vi "Teleop.vi"(10 "Match Info":T1={"Autonomous Elapsed Seconds"=0.0, "TeleOp Elapsed Seconds"=0.0, "Disabled Elapsed Seconds"=0.0, "Visited Autonomous"=FALSE, "Visited TeleOp"=FALSE, "Visited Disabled"=FALSE, "Autonomous Settings"={"Autonomous Style"=enum."Independent", "VI Refnum"=refnum}}, 11 "Call Context":T2) -> ()   [LabVIEW 2019]
doc: "This VI is called for each TeleOp packet received from the DS where the robot is not disabled. It is often used to read from the joysticks and update I/O or to update setpoints for timed control loops. It should complete and return within 20 milliseconds or it may miss DS packets."
uses:
  <vilib>/Rock Robotics/WPI/DriverStation/WPI_DriverStationDerivedRobotMode.ctl
  <vilib>/Rock Robotics/WPI/DriverStation/WPI_DriverStationMatch Info.ctl
  <vilib>/Rock Robotics/WPI/Utilities/WPI_GetSetVariantRefNum.vi
  <vilib>/Rock Robotics/Network Tables/NT Write Boolean Array.vi
  <vilib>/Rock Robotics/Network Tables/NT Write Numeric Array.vi
  <vilib>/Rock Robotics/Network Tables/NT Write Number.vi
  <vilib>/Rock Robotics/WPI/RobotDrive/WPI_RobotDriveMecanumDrive_Cartesian.vi
  <vilib>/Rock Robotics/WPI/RobotDrive/WPI_RobotDriveMecanumDrive_Polar.vi
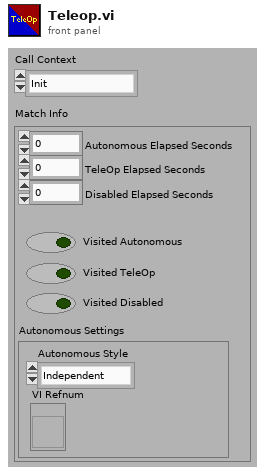
[diagram p1: front panel]
types:
  T1 = typedef "WPI_DriverStationMatch Info.ctl" = cluster{"Autonomous Elapsed Seconds":dbl, "TeleOp Elapsed Seconds":dbl, "Disabled Elapsed Seconds":dbl, "Visited Autonomous":bool, "Visited TeleOp":bool, "Visited Disabled":bool, "Autonomous Settings":cluster{"Autonomous Style":enum16{"Iterative", "Independent"}, "VI Refnum":refnum<vi>}}
  T2 = typedef "WPI_DriverStationDerivedRobotMode.ctl" = enum16{"Init", "Execute", "Stop"}
  T3 = typedef "WPI_JoystickDevRef.ctl" = cluster{"Device":T4}
  T4 = typedef "WPI_JoystickDeviceEnum.ctl" = enum16{"USB 0", "USB 1", "USB 2", "USB 3", "USB 4", "USB 5"}
  T5 = cluster{"Axes[0]":dbl, "Axes[1]":dbl, "Axes[2]":dbl, "Axes[3]":dbl, "Axes[4]":dbl, "Axes[5]":dbl, "Axes[6]":dbl, "Axes[7]":dbl, "Axes[8]":dbl}
  T6 = cluster{"Buttons[0]":bool, "Buttons[1]":bool, "Buttons[2]":bool, "Buttons[3]":bool, "Buttons[4]":bool, "Buttons[5]":bool, "Buttons[6]":bool, "Buttons[7]":bool, "Buttons[8]":bool, "Buttons[9]":bool, "Buttons[10]":bool, "Buttons[11]":bool}
  T7 = cluster{"Yaw":dbl, "Roll":dbl, "Pitch":dbl, "Heading":dbl, "Fused Heading":dbl}
  T8 = typedef "WPI_RobotDriveDevRef.ctl" = cluster{"DevStatus":errorcluster, "Motors[]":T9[], "Square Inputs":bool, "Max Output":dbl}
  T9 = typedef "WPI_MotorControlDeviceRef.ctl" = cluster{"DeviceStatus":errorcluster, "Type":T10, "PWM":cluster{"PWM Channel":T11, "DeadBand":T12}, "CAN":cluster{"Device Number":u8, "SetOutput VI Ref":variant, "GetOutput VI Ref":variant, "Enable VI Ref":variant, "Disable VI Ref":variant, "Data":variant}, "Invert":bool, "DIO PWM":cluster{"PWM \"Enable\" Channel":T11, "DIOChannel":T13, "PWM Rate":dbl}}
  T10 = typedef "WPI_MotorControlType.ctl" = enum16{"PWM", "CAN", "DIO PWM"}
  T11 = typedef "FPGA_DIOPWMChannel.ctl" = enum8{"PWM 0", "PWM 1", "PWM 2", "PWM 3", "PWM 4", "PWM 5", "PWM 6", "PWM 7", "PWM 8", "PWM 9", "PWM MXP 0", "PWM MXP 1", "PWM MXP 2", "PWM MXP 3", "PWM MXP 4", "PWM MXP 5", "PWM MXP 6", "PWM MXP 7", "PWM MXP 8", "PWM MXP 9", "Invalid"}
  T12 = typedef "WPI_PWMDeadband.ctl" = cluster{"Name":string, "maxPositivePwm":i32, "minPositivePwm":i32, "centerPwm":i32, "maxNegativePwm":i32, "minNegativePwm":i32, "angularRange":u16}
  T13 = typedef "FPGA_DIOChannel.ctl" = enum8{"DIO 0", "DIO 1", "DIO 2", "DIO 3", "DIO 4", "DIO 5", "DIO 6", "DIO 7", "DIO 8", "DIO 9", "DIO MXP 0", "DIO MXP 1", "DIO MXP 2", "DIO MXP 3", "DIO MXP 4", "DIO MXP 5", "DIO MXP 6", "DIO MXP 7", "DIO MXP 8", "DIO MXP 9", "DIO MXP 10", "DIO MXP 11", "DIO MXP 12", "DIO MXP 13", "DIO MXP 14", "DIO MXP 15", "SPI Port CS1", "SPI Port CS2", "SPI Port CS3", "SPI Port MISO", "SPI Port MOSI", "Invalid"}
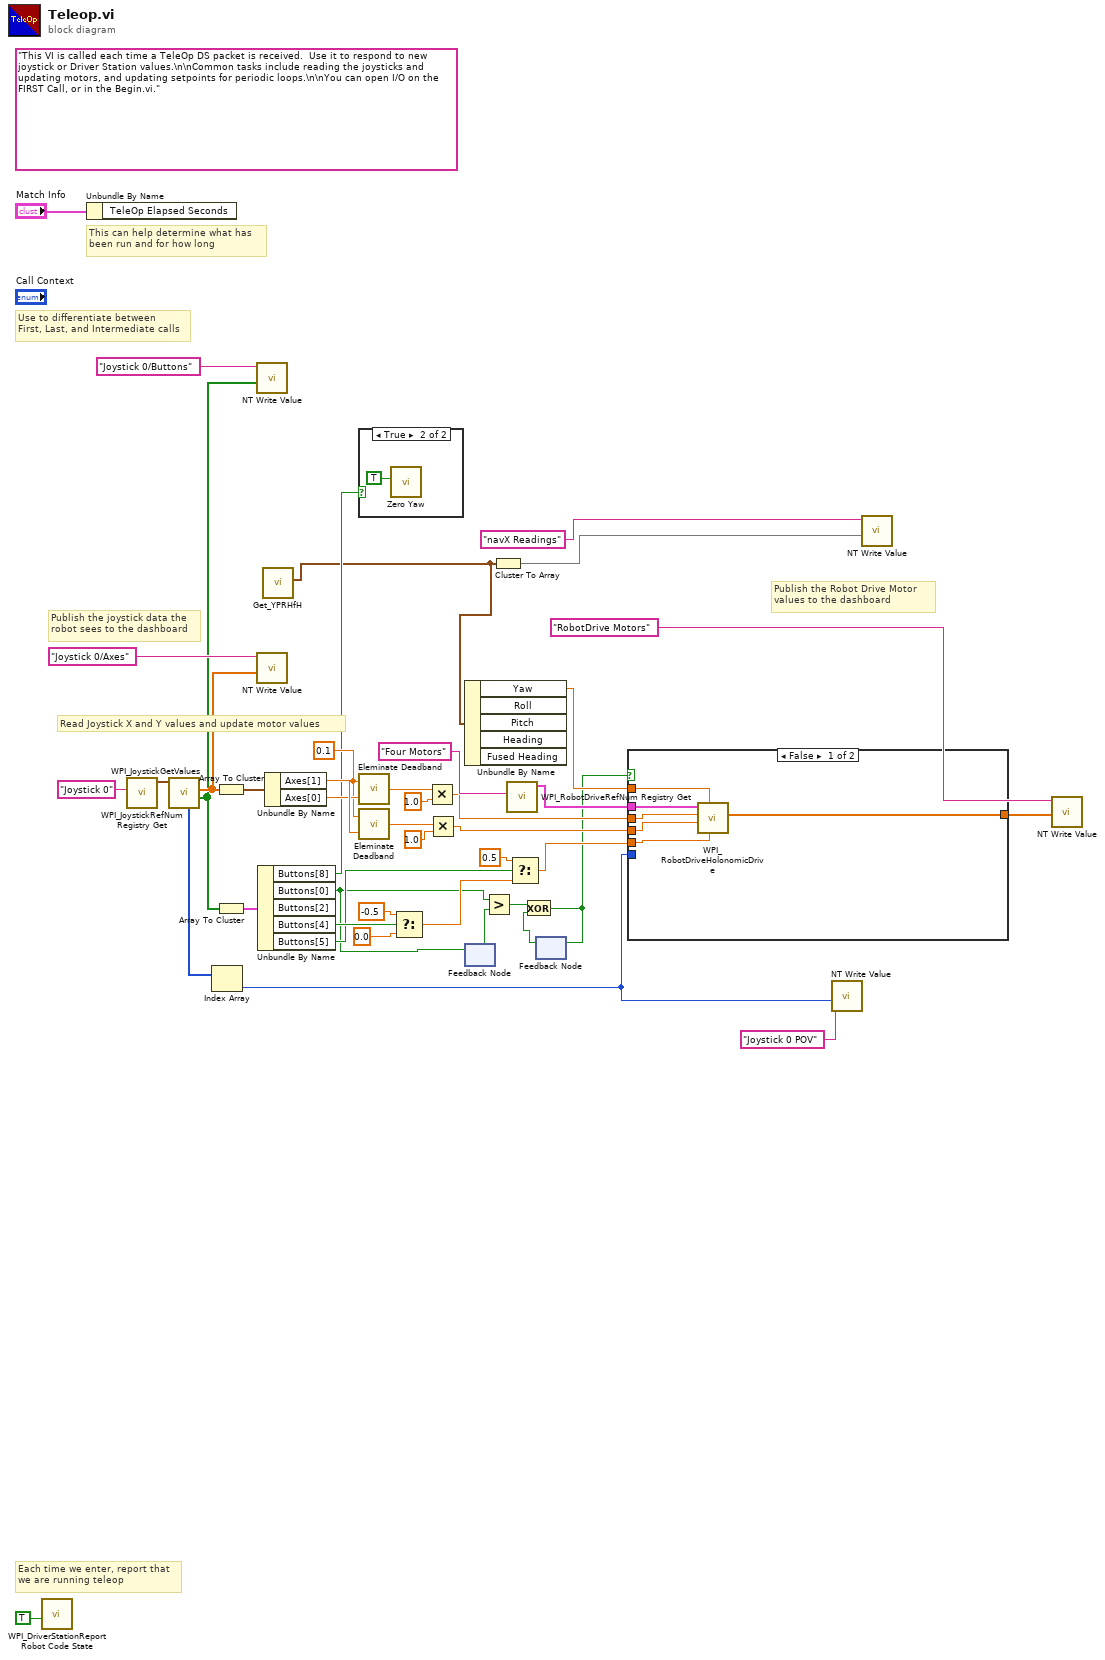
[diagram p0: block diagram]
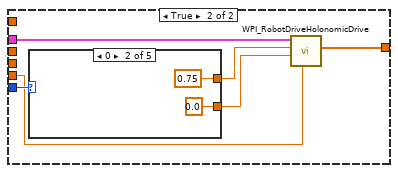
[diagram p2: hidden frame]
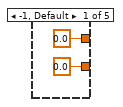
[diagram p3: hidden frame]
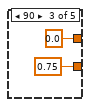
[diagram p4: hidden frame]
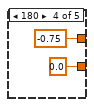
[diagram p5: hidden frame]
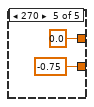
[diagram p6: hidden frame]
diagram:
  w27 = 0.1 ("Deadband")
  (unwired) "This VI is called each time a TeleOp DS packet is received.  Use it to respond to new joystick or Driver Station values.\n\nCommon tasks include reading the joysticks and updating motors, and updating setpoints for periodic loops.\n\nYou can open I/O on the FIRST Call, or in the Begin.vi."
  # "Publish the Robot Drive Motor\nvalues to the dashboard"
  # "Publish the joystick data the\nrobot sees to the dashboard"
  # "Each time we enter, report that\nwe are running teleop"
  # "Use to differentiate between\nFirst, Last, and Intermediate calls"
  # "This can help determine what has\nbeen run and for how long"
  # "Read Joystick X and Y values and update motor values"
  n1 = call <vilib>:"WPI_DriverStationReport Robot Code State.vi"("TeleOp"=TRUE ("Autonomous")) -> ()  [unwired: 10 in, 1 out]
  n2 = Unbundle By Name("Match Info") -> ()  [unwired: 1 out]
  n3 = call <vilib>:"WPI_JoystickRefNum Registry Get.vi"("refnum name"="Joystick 0") -> ("JoystickDevRef"=w39:T3)  [unwired: 1 in, 9 out]
  n4 = call <vilib>:"WPI_JoystickGetValues.vi"("JoystickDevRef"=w39) -> ("Buttons"=w30:bool[], "Axes"=w33:dbl[], "POVs"=w9:i16[])  [unwired: 6 in, 2 out]
  n5 = Index Array(array=w9) -> (element=w2:i16)  [unwired: 1 in]
  n6 = Array To Cluster(array=w33) -> (cluster=w32:T5)
  n7 = Array To Cluster(array=w30) -> (cluster=w31:T6)
  n8 = call-poly <vilib>:"NT Write Value.vi"("Boolean Array"=w30, "Name"="Joystick 0/Buttons") -> ()  [unwired: 9 in, 1 out]
  n9 = call-poly <vilib>:"NT Write Value.vi"("Numeric Array"=w33, "Name"="Joystick 0/Axes") -> ()  [unwired: 9 in, 1 out]
  n10 = Unbundle By Name(w31) -> ("Buttons[8]"=w26:bool, "Buttons[0]"=w4:bool, "Buttons[4]"=w18:bool, "Buttons[5]"=w17:bool)  [unwired: 1 out]
  n11 = call <vilib>:"Get_YPRHfH.vi"() -> ("YRPHfH"=w1:T7)  [unwired: 11 in]
  n12 = Unbundle By Name(w32) -> ("Axes[1]"=w29:dbl, "Axes[0]"=w28:dbl)
  n13 = case shown="True" w26 {
    frame False {
    }
    frame True {
      n14 = call <vilib>:"Zero Yaw.vi"("Zero"=TRUE) -> ()  [unwired: 11 in]
    }
  }
  n15 = call "Eleminate Deadband.vi"("Axis In"=w28, "Deadband"=w27) -> ("Axis Out"=w14:dbl)
  n16 = call "Eleminate Deadband.vi"("Axis In"=w29, "Deadband"=w27) -> ("Axis Out"=w11:dbl)
  n17 = Select(t=-0.5, s=w18, f=0.0) -> (s? t:f=w22:dbl)
  n18 = Multiply(x=w14, y=1.0) -> (x*y=w15:dbl)
  n19 = Multiply(x=w11, y=1.0) -> (x*y=w12:dbl)
  n20 = Unbundle By Name(w1) -> ("Yaw"=w25:dbl)  [unwired: 4 out]
  n21 = feedback #1() -> (w5:bool)  [unwired: 1 in]
  n22 = feedback-in #1(w4) -> ()
  n23 = Greater?(x=w4, y=w5) -> (0:w6:bool)
  n24 = Cluster To Array(cluster=w1) -> (array=w23:dbl[])
  n25 = call <vilib>:"WPI_RobotDriveRefNum Registry Get.vi"("refnum name"="Four Motors") -> ("RobotDriveDevRef"=w41:T8)  [unwired: 1 in, 9 out]
  n26 = Select(t=0.5, s=w17, f=w22) -> (s? t:f=w16:dbl)
  n27 = feedback #2() -> (w7:bool)  [unwired: 1 in]
  n28 = Exclusive Or(1:w7, 2:w6) -> (0:w8:bool)
  n29 = feedback-in #2(w8) -> ()
  n30 = case shown="False" w8 {
    tunnel: w41 -> [w50 w55]
    tunnel: [w49 w56] -> w35
    tunnel: w25 -> [w45 _]
    tunnel: w16 -> [w48 w53]
    tunnel: w15 -> [w47 _]
    tunnel: w12 -> [w46 _]
    tunnel: w2 -> [_ w54]
    frame False {
      n31 = call-poly <vilib>:"WPI_RobotDriveHolonomicDrive.vi"("Rotation"=w48, "Gyro Angle"=w45, "Y"=w46, "X"=w47, "RobotDriveDevRef"=w50) -> ("Motor Values"=w49:dbl[])  [unwired: 4 in, 2 out]
    }
    frame True {
      n32 = case shown="0" w54 {
        tunnel: [0.0 0.75 0.0 -0.75 0.0] -> w52
        tunnel: [0.0 0.0 0.75 0.0 -0.75] -> w51
        frame -1, Default {
        }
        frame 0 {
        }
        frame 90 {
        }
        frame 180 {
        }
        frame 270 {
        }
      }
      n33 = call-poly <vilib>:"WPI_RobotDriveHolonomicDrive.vi"("Rotation"=w53, "Direction"=w51, "Magnitude"=w52, "RobotDriveDevRef"=w55) -> ("Motor Values"=w56:dbl[])  [unwired: 5 in, 2 out]
    }
  }
  n34 = call-poly <vilib>:"NT Write Value.vi"("Numeric"=w2, "Name"="Joystick 0 POV") -> ()  [unwired: 9 in, 1 out]
  n35 = call-poly <vilib>:"NT Write Value.vi"("Numeric Array"=w23, "Name"="navX Readings") -> ()  [unwired: 9 in, 1 out]
  n36 = call-poly <vilib>:"NT Write Value.vi"("Numeric Array"=w35, "Name"="RobotDrive Motors") -> ()  [unwired: 9 in, 1 out]
